vi "Get Map calib transform coeffs_PN.vi"(0 "B1 from Vel. Calib":dbl=1.36, 1 "A1 from Vel. Calib":dbl=2.21, 5 "n1 from Vel. Calib":dbl=0.42, 7 "Zero angle dataset from map (used for calib. correction)":dbl[][](array[numeric]), 9 "A2 from Vel. Calib":dbl=2.25, 11 "B2 from Vel. Calib":dbl=1.4, 12 "n2 from Vel. Calib":dbl=0.41) -> (4 "S*cos(q), S*sin(q), Tx, Ty":dbl[](array[numeric])=[1.0763223002323654, 0.0007524070719776288, -0.14779165640104555, -0.09827403757225917], 6 "Sx, Tx, Sy, Ty":dbl[](array[numeric])=[1.0000263372329348, -5.817138285027323e-05, 0.9999727510054321, 6.062261811624134e-05], 10 "Mean % rel. err in E1'":dbl=0.13306717681825547 format="%_3g", 15 "Mean % rel. err in E2'":dbl=0.17334903746251706 format="%_3g")   [LabVIEW 2010]
uses:
  <vilib>/Analysis/Matrix/Numeric/Conversions/Array To Matrix - RA.vi
  <vilib>/Analysis/Matrix/Numeric/Conversions/Array To Matrix - RA2.vi
  <vilib>/Analysis/7linalg.llb/Solve Linear Equations (multiple right hand).vi
  <vilib>/Analysis/Matrix/Numeric/Conversions/Matrix To Array - RM.vi
  <vilib>/Analysis/baseanly.llb/A x Vector.vi
  <vilib>/Analysis/NI_AALPro.lvlib
  <vilib>/Analysis/Matrix/NI_Matrix.lvlib
  <vilib>/Analysis/NI_AALBase.lvlib
panel:
  out "E1, E2 corrected and un-corrected against calib.":T1(graph)
  out "Std. dev in % rel. err in E2'":dbl=0.1720370852263028 format="%_3g"
  out "Max % rel. err in E2'":dbl=0.6224424154220581 format="%#_3g"
  out "Min % rel. err in E2'":dbl=0.007548057269662263 format="%#_3g"
  out "Min % rel. err in E1'":dbl=0.01033569515821781 format="%#_3g"
  out "Max % rel. err in E1'":dbl=0.5570184231617936 format="%#_3g"
  out "Std. dev in % rel. err in E1'":dbl=0.1606948404137527 format="%_3g"
  out "E1' uSRT --> ST":dbl[](array[numeric])=[1.815892021046585, 1.8849009507024945, 2.001924270772093, 2.086318145030956, 2.1535433895702463, 2.209179886740718, 2.29997211446669, 2.373957582009073, 2.436794150450389, 2.491940391006859, 2.5414176269987556]
  out "E2' uSRT --> ST":dbl[](array[numeric])=[1.8385583017101361, 1.9097387773209844, 2.021749720792284, 2.1027675103611636, 2.1689581187863016, 2.2235973787283823, 2.31310621507788, 2.3865557671816875, 2.4493045501265316, 2.5040672411234945, 2.5540149374604875]
  out "E2' uSRT":dbl[](array[numeric])=[1.8385477776704264, 1.9097301929305215, 2.0217441886705823, 2.102764185952928, 2.1689565980547436, 2.223597346902293, 2.313108622344049, 2.386560175928841, 2.4493106687615236, 2.5040748520274185, 2.5540239094260055]
  out "E1' uSRT":dbl[](array[numeric])=[1.8159023665858196, 1.884909478785341, 2.0019297168656713, 2.086321368481948, 2.153544842540943, 2.2091798744386204, 2.299969711011518, 2.3739532300327273, 2.436788143576289, 2.4919329317716272, 2.5414088647043536]
  out "Map uniform scale fact.":dbl=1.0763225632187163
  out "Map rot (deg)":dbl=0.040052819372575564
  # "Paul Nathan 16/02/10"
  # "Transformation equations given below"
  # "First apply uniform scaling with rotation and translation:"
  # "then apply independent scaling with translation onto the points mapped with the above transformation (as a final correction, typically small)"
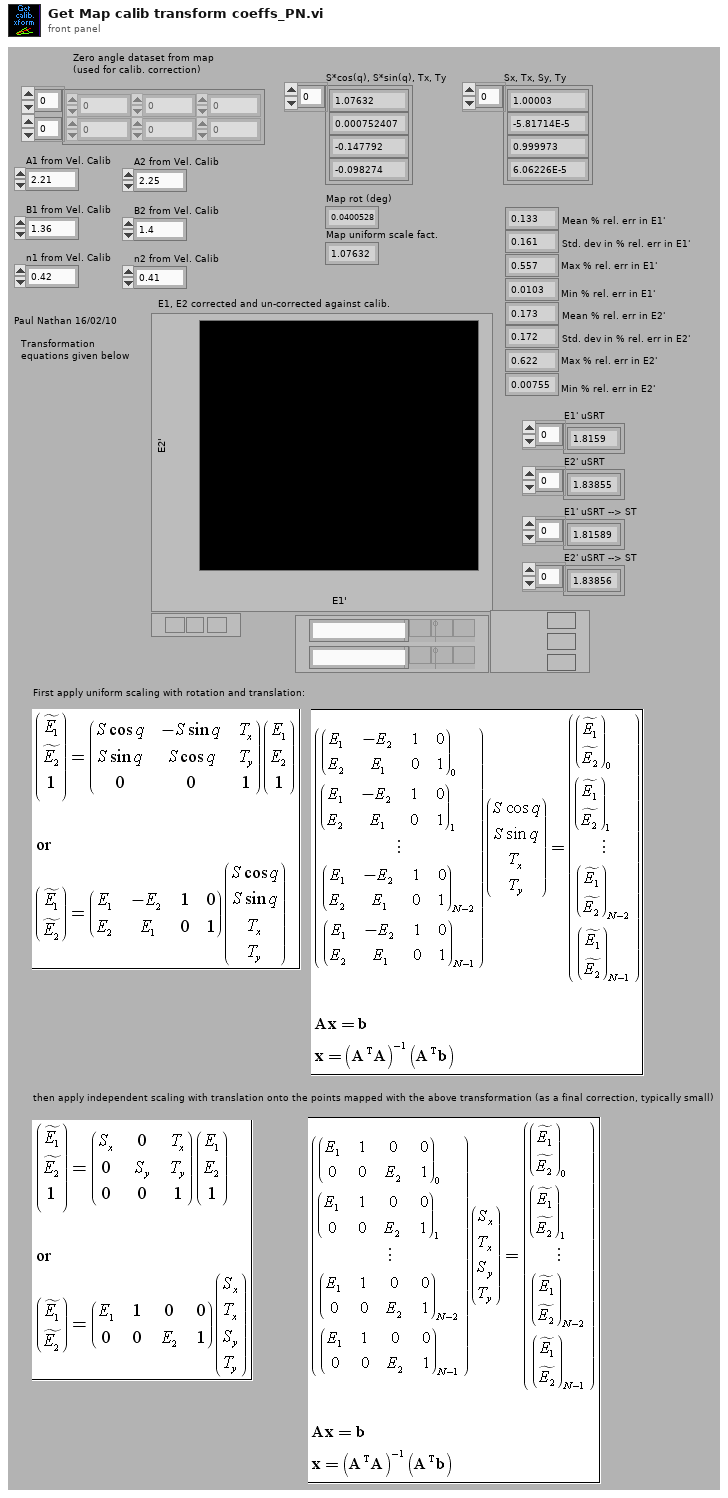
[diagram p1: front panel]
types:
  T1 = cluster{"Zero angle dataset from map (used for calib. correction)":dbl[], "Zero angle dataset from map (used for calib. correction)":dbl[]}[]
  T2 = cluster{"Zero angle dataset from map (used for calib. correction)":dbl[], "Zero angle dataset from map (used for calib. correction)":dbl[]}
  T3 = typedef "NI_Matrix.lvlib/RealMatrix.ctl" = dbl[][]
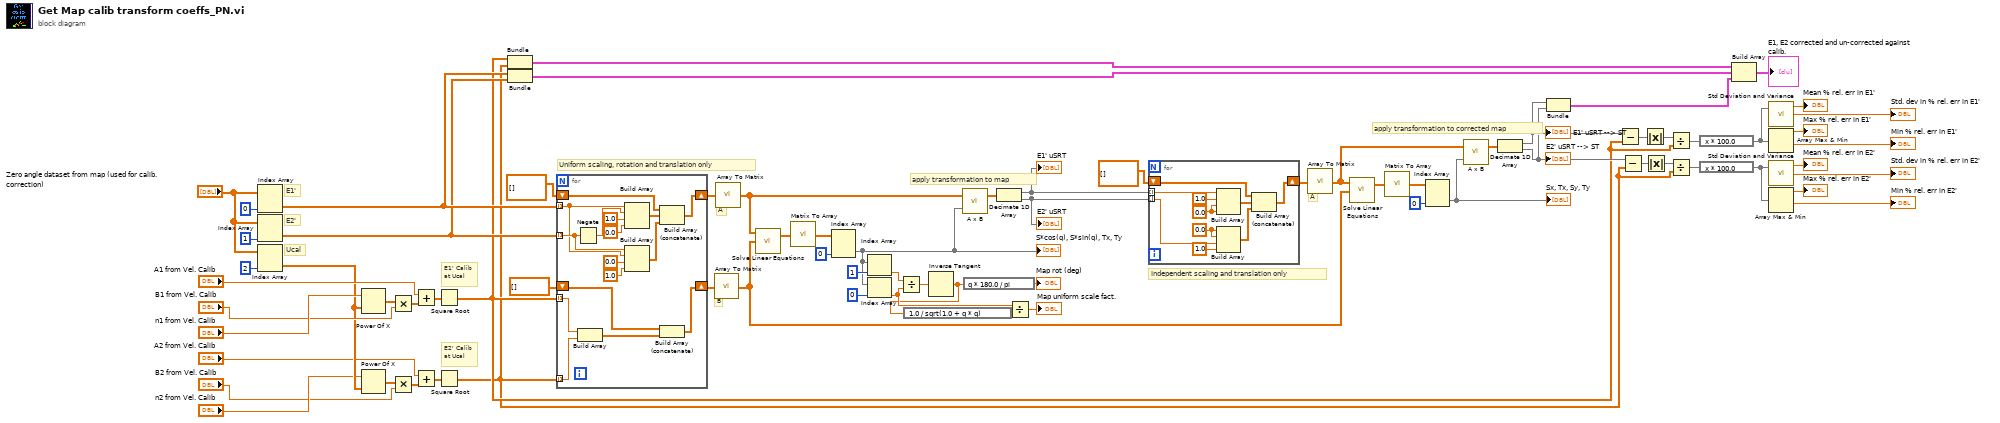
[diagram p0: block diagram]
diagram:
  # "apply transformation to corrected map"
  # "apply transformation to map"
  # "Independent scaling and translation only"
  # "Uniform scaling, rotation and translation only"
  # "E2' Calib at Ucal"
  # "A"
  # "A"
  # "B"
  # "E1' Calib at Ucal"
  # "Ucal"
  # "E2'"
  # "E1'"
  n1 = Index Array(array="Zero angle dataset from map (used for calib. correction)", index (col)=0 ("disabled index (col)")) -> (element=w9:dbl[])  [unwired: 1 in]
  n2 = Index Array(array="Zero angle dataset from map (used for calib. correction)", index (col)=1 ("disabled index (col)")) -> (element=w8:dbl[])  [unwired: 1 in]
  n3 = Index Array(array="Zero angle dataset from map (used for calib. correction)", index (col)=2 ("disabled index (col)")) -> (element=w61:dbl[])  [unwired: 1 in]
  n4 = Power Of X(1:w61, 2:"n1 from Vel. Calib") -> (0:w69:dbl[])
  n5 = Power Of X(1:w61, 2:"n2 from Vel. Calib") -> (0:w62:dbl[])
  n6 = Multiply(x=w69, y="B1 from Vel. Calib") -> (x*y=w66:dbl[])
  n7 = Multiply(x=w62, y="B2 from Vel. Calib") -> (x*y=w63:dbl[])
  n8 = Add(x="A1 from Vel. Calib", y=w66) -> (x+y=w65:dbl[])
  n9 = Add(x="A2 from Vel. Calib", y=w63) -> (x+y=w64:dbl[])
  n10 = Square Root(x=w65) -> (sqrt(x)=w7:dbl[])
  n11 = Square Root(x=w64) -> (sqrt(x)=w6:dbl[])
  n12 = Bundle(w7, w6) -> (w5:cluster{dbl[], dbl[]})  [unwired: 1 out]
  n13 = Bundle("Zero angle dataset from map (used for calib. correction)"=w9, "Zero angle dataset from map (used for calib. correction)"=w8) -> (w4:T2)  [unwired: 1 out]
  n14 = for {
    tunnel: w9 -> [w83] mode=indexing
    tunnel: w8 -> [w84] mode=indexing
    tunnel: w7 -> [w78] mode=indexing
    tunnel: w6 -> [w77] mode=indexing
    shift-right: [w82] -> w37
    shift-left: dbl[][] [] -> [w81]
    shift-right: [w76] -> w56
    shift-left: dbl[] [] -> [w74]
    n15 = Negate(x=w84) -> (-x=w89:dbl)
    n16 = Build Array(w78, w77) -> (w75:dbl[])
    n17 = Build Array(w83, w89, 1.0 ("element"), 0.0 ("element")) -> (w80:dbl[])
    n18 = Build Array(w84, w83, 0.0 ("element"), 1.0 ("element")) -> (w79:dbl[])
    n19 = Build Array (concatenate)(w81, w80, w79) -> (w82:dbl[][])
    n20 = Build Array (concatenate)(w74, w75) -> (w76:dbl[])
  }
  n21 = call-poly <vilib>:"Array To Matrix.vi"("Real 1D Array"=w56) -> ("Real Matrix (Column Vector)"=w31:T3)
  n22 = call-poly <vilib>:"Array To Matrix.vi"("Real 2D Array"=w37) -> ("Real Matrix"=w36:T3)
  n23 = call-poly <vilib>:"Solve Linear Equations.vi"("Known Matrix"=w31, "Input Matrix"=w36) -> ("Solution Matrix"=w54:T3)  [unwired: 1 in, 1 out]
  n24 = call-poly <vilib>:"Matrix To Array.vi"("Real Matrix"=w54) -> ("Real 2D Array"=w53:dbl[][])
  n25 = Index Array(array=w53, index (col)=0 ("index (row)")) -> (element=w35:dbl[])  [unwired: 1 in]
  "S*cos(q), S*sin(q), Tx, Ty" <- w35
  n26 = Index Array(array=w35, index=1 ("index (row)")) -> (element=w44:dbl)
  n27 = Index Array(array=w35, index=0 ("index (row)")) -> (element=w41:dbl)
  n28 = Divide(x=w44, y=w41) -> (x/y=w43:dbl)
  n29 = Inverse Tangent(1:w43) -> (0:w40:dbl)
  n30 = expression code="1.0 / sqrt(1.0 + q * q)"(w40) -> (w39:dbl)
  n31 = call-poly <vilib>:"A x B.vi"("Vector"=w35, "A"=w36) -> ("A x Vector"=w34:dbl[])  [unwired: 1 out]
  n32 = expression code="q * 180.0 / pi"(w40) -> (→"Map rot (deg)":dbl)
  n33 = Decimate 1D Array(w34) -> (w32:dbl[], w33:dbl[])
  "E1' uSRT" <- w32
  "E2' uSRT" <- w33
  n34 = Divide(x=w41, y=w39) -> (x/y=→"Map uniform scale fact.":dbl)
  n35 = for {
    tunnel: w32 -> [w98] mode=indexing
    tunnel: w33 -> [w92] mode=indexing
    shift-right: [w97] -> w50
    shift-left: dbl[][] [] -> [w96]
    w90 = 0.0 ("element")
    w91 = 0.0 ("element")
    n36 = Build Array(w98, 1.0 ("element"), w91, w91) -> (w95:dbl[])
    n37 = Build Array(w90, w90, w92, 1.0 ("element")) -> (w94:dbl[])
    n38 = Build Array (concatenate)(w96, w95, w94) -> (w97:dbl[][])
  }
  n39 = call-poly <vilib>:"Array To Matrix.vi"("Real 2D Array"=w50) -> ("Real Matrix"=w30:T3)
  n40 = call-poly <vilib>:"Solve Linear Equations.vi"("Known Matrix"=w31, "Input Matrix"=w30) -> ("Solution Matrix"=w51:T3)  [unwired: 1 in, 1 out]
  n41 = call-poly <vilib>:"Matrix To Array.vi"("Real Matrix"=w51) -> ("Real 2D Array"=w52:dbl[][])
  n42 = Index Array(array=w52, index (col)=0 ("index (row)")) -> (element=w29:dbl[])  [unwired: 1 in]
  "Sx, Tx, Sy, Ty" <- w29
  n43 = call-poly <vilib>:"A x B.vi"("Vector"=w29, "A"=w30) -> ("A x Vector"=w28:dbl[])  [unwired: 1 out]
  n44 = Decimate 1D Array(w28) -> (w11:dbl[], w10:dbl[])
  "E1' uSRT --> ST" <- w11
  "E2' uSRT --> ST" <- w10
  n45 = Bundle(w11, w10) -> (w3:cluster{dbl[], dbl[]})  [unwired: 1 out]
  n46 = Subtract(x=w11, y=w7) -> (x-y=w27:dbl[])
  n47 = Subtract(x=w10, y=w6) -> (x-y=w26:dbl[])
  n48 = Absolute Value(x=w27) -> (abs(x)=w21:dbl[])
  n49 = Absolute Value(x=w26) -> (abs(x)=w12:dbl[])
  n50 = Divide(x=w21, y=w7) -> (x/y=w20:dbl[])
  n51 = Divide(x=w12, y=w6) -> (x/y=w17:dbl[])
  n52 = expression code="x * 100.0"(w20) -> (w19:dbl[])
  n53 = expression code="x * 100.0"(w17) -> (w18:dbl[])
  n54 = Build Array(w5, w4, w3) -> (→"E1, E2 corrected and un-corrected against calib.":T1)
  n55 = call <vilib>:"Std Deviation and Variance.vi"("X"=w19) -> ("mean"=→"Mean % rel. err in E1'":dbl, "standard deviation"=→"Std. dev in % rel. err in E1'":dbl)  [unwired: 1 in, 1 out]
  n56 = Array Max & Min(array=w19) -> (max value=→"Max % rel. err in E1'":dbl, min value=→"Min % rel. err in E1'":dbl)  [unwired: 2 out]
  n57 = call <vilib>:"Std Deviation and Variance.vi"("X"=w18) -> ("mean"=→"Mean % rel. err in E2'":dbl, "standard deviation"=→"Std. dev in % rel. err in E2'":dbl)  [unwired: 1 in, 1 out]
  n58 = Array Max & Min(array=w18) -> (max value=→"Max % rel. err in E2'":dbl, min value=→"Min % rel. err in E2'":dbl)  [unwired: 2 out]
